vi "MSGR Tree.vi"   [LabVIEW 2018]
doc: "MIT License\n\nCopyright (c) 2020 RichardLGP5\n\nPermission is hereby granted, free of charge, to any person obtaining a copy\nof this software and associated documentation files (the \"Software\"), to deal\nin the Software without restriction, including without limitation the rights\nto use, copy, modify, merge, publish, distribute, sublicense, and/or sell\ncopies of the Software, and to permit persons to whom the Software is\nfurnished to do so, subject to the following conditions:\n\nThe above copyright notice and this permission notice shall be included in all\ncopies or substantial portions of the Software.\n\nTHE SOFTWARE IS PROVIDED \"AS IS\", WITHOUT WARRANTY OF ANY KIND, EXPRESS OR\nIMPLIED, INCLUDING BUT NOT LIMITED TO THE WARRANTIES OF MERCHANTABILITY,\nFITNESS FOR A PARTICULAR PURPOSE AND NONINFRINGEMENT. IN NO EVENT SHALL THE\nAUTHORS OR COPYRIGHT HOLDERS BE LIABLE FOR ANY CLAIM, DAMAGES OR OTHER\nLIABILITY, WHETHER IN AN ACTION OF CONTRACT, TORT OR OTHERWISE, ARISING FROM,\nOUT OF OR IN CONNECTION WITH THE SOFTWARE OR THE USE OR OTHER DEALINGS IN THE\nSOFTWARE."
uses:
  MSGR Q Data TypeDef.ctl
types:
  T1 = typedef "MSGR Q Data TypeDef.ctl" = cluster{"Msg":string, "Parameters":string, "Reply?":bool, "ReplyQ":string}
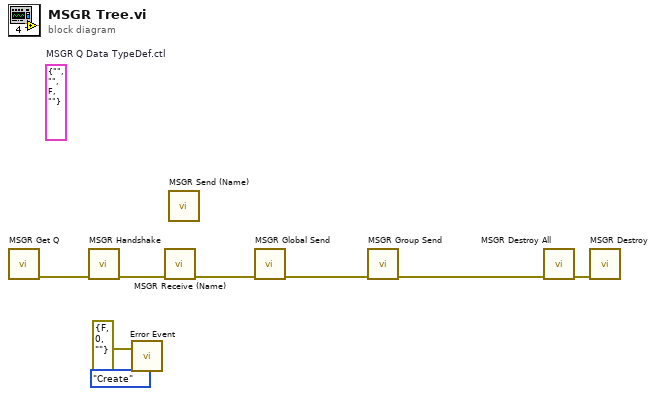
[diagram p0: block diagram]
diagram:
  (unwired) T1 {"Msg"="", "Parameters"="", "Reply?"=FALSE, "ReplyQ"=""}  # MSGR Q Data TypeDef.ctl
  n1 = call "MSGR Get Q.vi"() -> ("error out"=w8:errorcluster)  [unwired: 10 in, 1 out]
  n2 = call "MSGR Handshake.vi"("error in (no error)"=w8) -> ("error out"=w7:errorcluster)  [unwired: 12 in, 2 out]
  n3 = call "Error Event.vi"("error in (no error)"=errorcluster {"status"=FALSE, "code"=0, "source"=""}, "Enum"=enum16{"Create", "Default", "Destroy"}."Create") -> ()  [unwired: 4 in, 2 out]
  n4 = call "MSGR Receive (Name).vi"("error in (no error)"=w7) -> ("error out"=w6:errorcluster)  [unwired: 12 in, 2 out]
  n5 = call "MSGR Send (Name).vi"() -> ()  [unwired: 14 in, 2 out]
  n6 = call "MSGR Global Send.vi"("error in (no error)"=w6) -> ("error out"=w5:errorcluster)  [unwired: 13 in, 1 out]
  n7 = call "MSGR Group Send.vi"("error in (no error)"=w5) -> ("error out"=w4:errorcluster)  [unwired: 13 in, 1 out]
  n8 = call "MSGR Destroy All.vi"("error in (no error)"=w4) -> ("error out"=w3:errorcluster)  [unwired: 14 in]
  n9 = call "MSGR Destroy.vi"("error in (no error)"=w3) -> ()  [unwired: 14 in, 1 out]
